vi "WallFollowV4.vi"(4 "Instruction Number":dbl=1.0 format="%#_13g", 6 "Speed Multuiplier":dbl=1.0 format="%#_13g", 7 "Estimated Distnace Travelled (mm)":dbl, 8 "Instruction":T4={"Direction"=enum."Forward", "Relative Tracked Wall"=enum."CW", "Tracking Distance (mm)"=0.0, "Relative Stop Direction"=enum."Dir. of travel", "Stop Distance (mm)"=0.0, "Forward Speed"=0.0, "Action"=enum."None", "Movement"=enum."Normal", "Zone (mm)"=300.0, "Lidar Detection Distance"=300.0}, 9 "Valid":bool[](array[boolean]), 10 "Lidar Angles (deg)":dbl[](array[numeric]), 11 "Lidar Distances (mm)":dbl[](array[numeric])) -> (0 "Direction":T3, 1 "Rotation":dbl, 2 "left/Right":dbl, 3 "Forward/Back":dbl, 5 "Motion Complete":bool)   [LabVIEW 2014]
uses:
  Types/Instruction.ctl
  Types/Direction.ctl
  Types/Action.ctl
  Types/Movement.ctl
panel:
  out "Zone (mm)":dbl
  out "Movement":T1
  out "Relative Tracked Wall":enum16{"None", "CW", "CCW"}(ring)
  out "Mean Distance":dbl[](array[numeric])
  out "Forward Speed (Specified)":dbl
  out "Forward Speed (Clamped)":dbl
  out "Forward Speed (Mult)":dbl
  out "Motor Speed (Chart)":dbl(graph)
  out "Relative Stop Direction":T2(ring)
  out "Left":dbl(slide)
  out "Right":dbl(slide) scale=0.0..500.0
  out "Back":dbl(slide) scale=500.0..0.5
  out "Front":dbl(slide) scale=0.0..500.0
  out "Tracking Distance (mm)":dbl
  out "Stop Distance (mm)":dbl
  out "Forward Speed":dbl
  out "Rotation Speed (Chart)":dbl(graph)
  out "Stop Wall Error":dbl
  out "Wall Rotation Error":dbl
  out "Wall Tracking Error":dbl
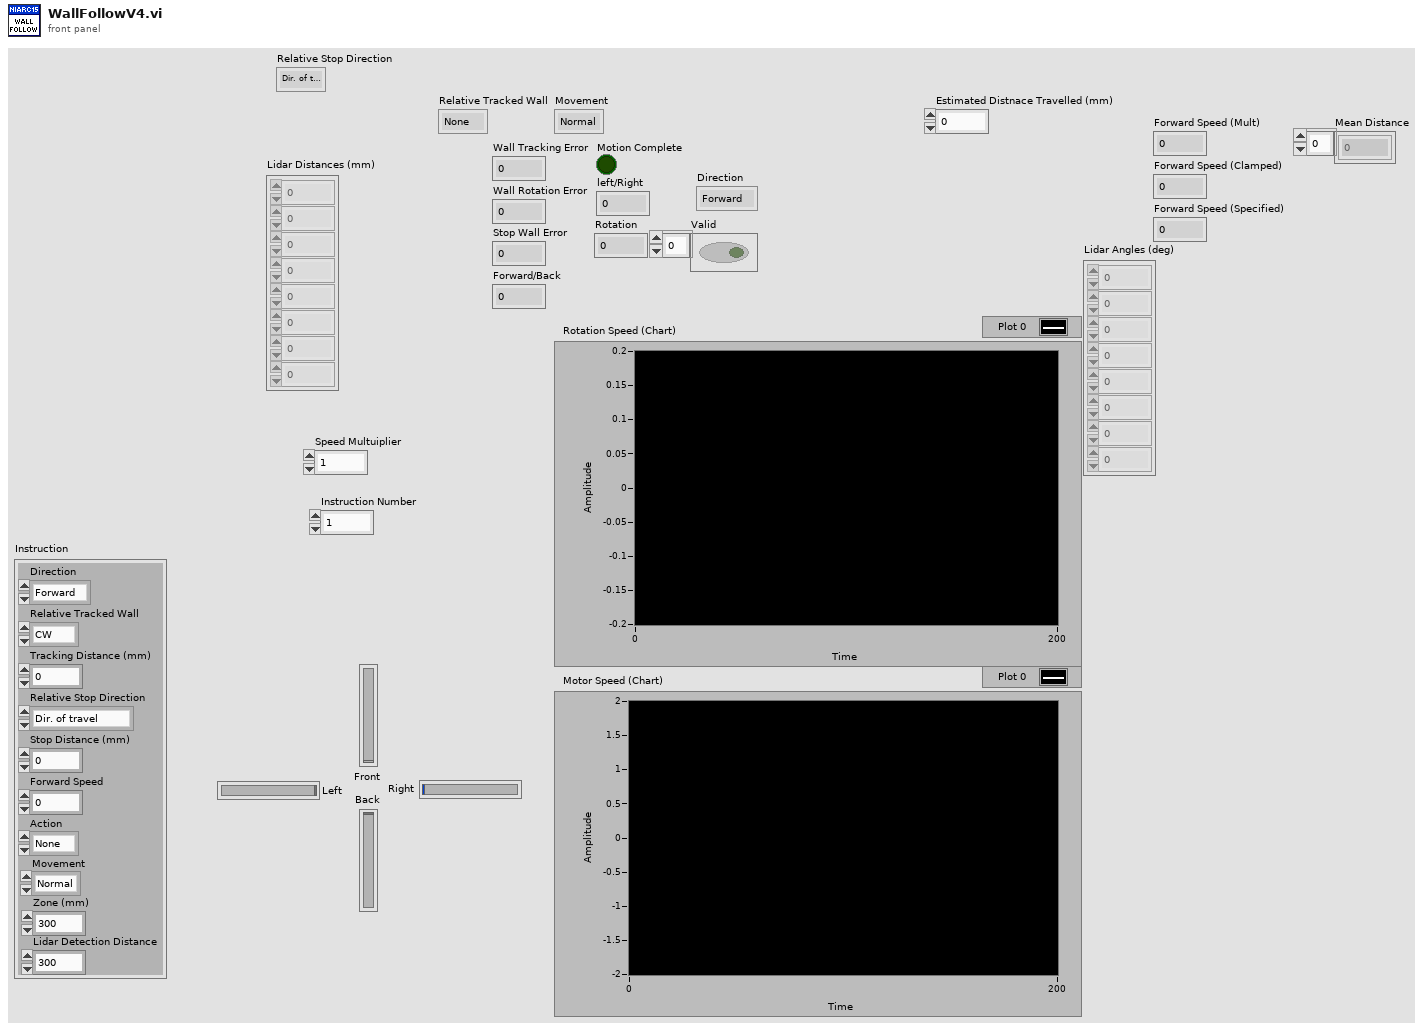
[diagram p1: front panel]
types:
  T1 = typedef "Movement.ctl" = enum16{"Normal", "Align", "Front Right", "Back Right"}
  T2 = enum16{"Dir. of travel", "Counter-dir of travel", "Distance"}
  T3 = typedef "Direction.ctl" = enum16{"Forward", "Left", "Back", "Right"}
  T4 = typedef "Instruction.ctl" = cluster{"Direction":T3, "Relative Tracked Wall":enum16{"None", "CW", "CCW"}, "Tracking Distance (mm)":dbl, "Relative Stop Direction":enum16{"Dir. of travel", "Counter-dir of travel", "Distance"}, "Stop Distance (mm)":dbl, "Forward Speed":dbl, "Action":T5, "Movement":T1, "Zone (mm)":dbl, "Lidar Detection Distance":dbl}
  T5 = typedef "Action.ctl" = enum16{"None", "Wait for Go", "Drop B", "Drop A", "Drop C", "Drop Rear"}
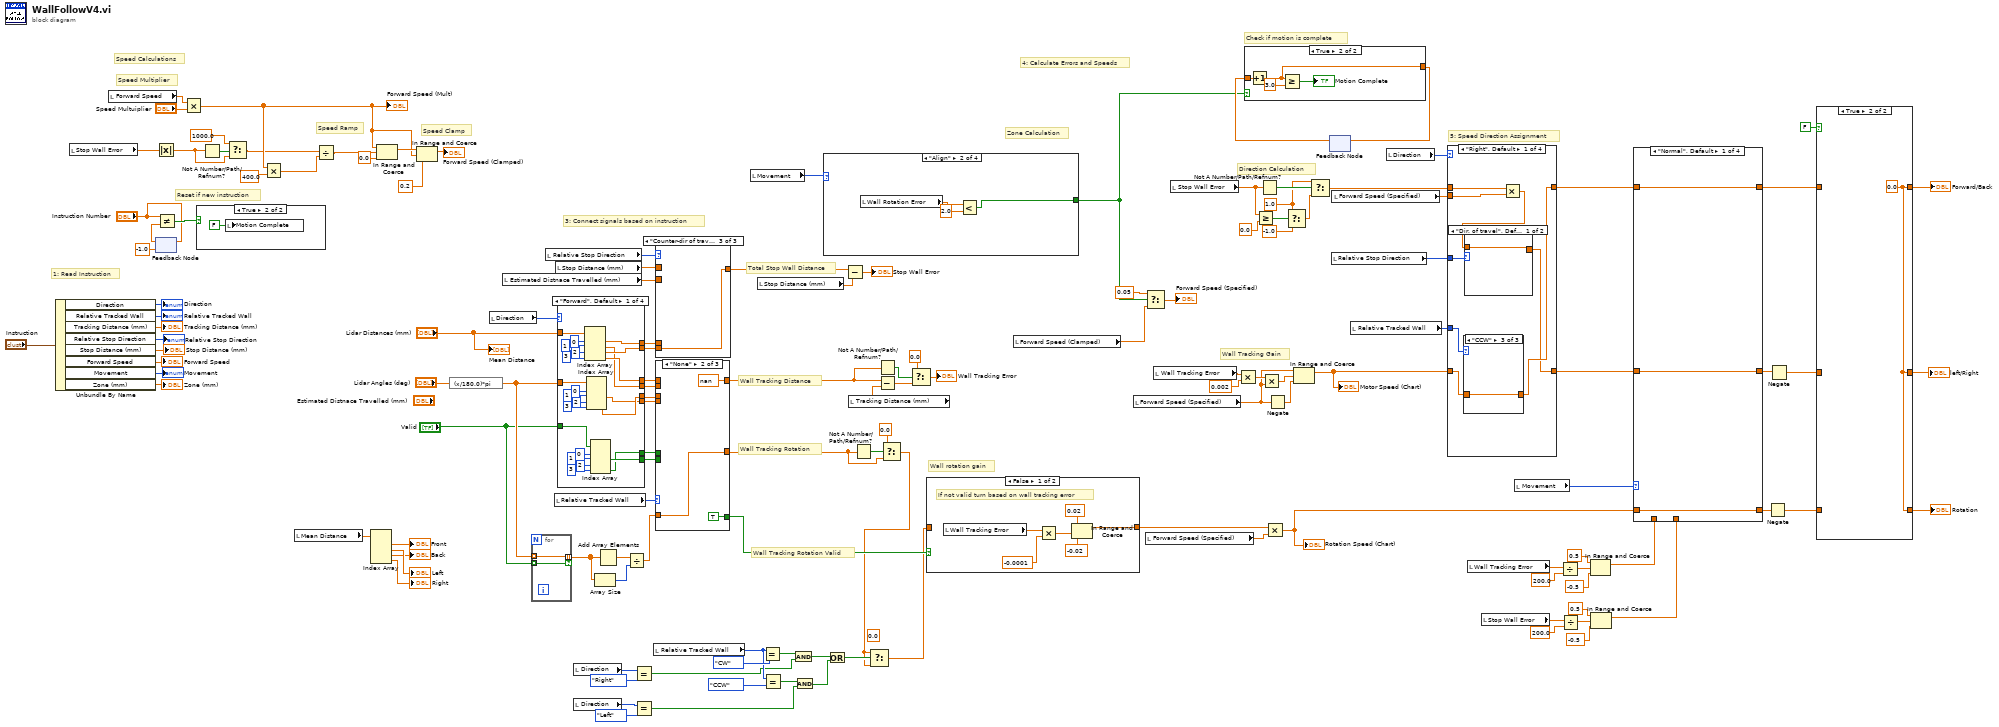
[diagram p0: block diagram]
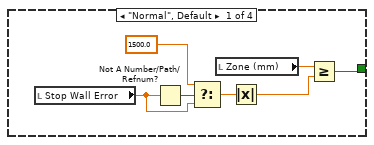
[diagram p4: hidden frame]
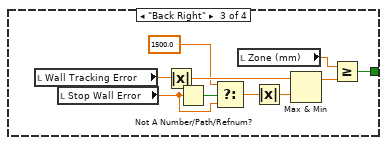
[diagram p5: hidden frame]
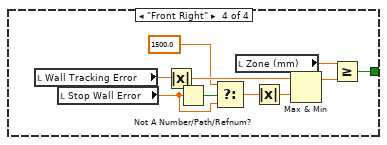
[diagram p6: hidden frame]
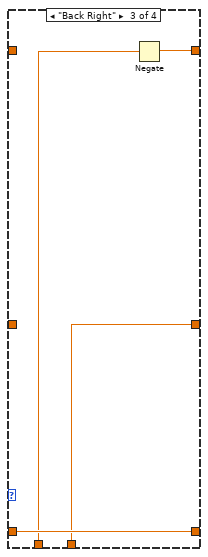
[diagram p8: hidden frame]
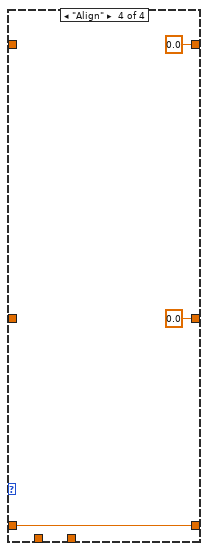
[diagram p9: hidden frame]
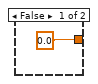
[diagram p10: hidden frame]
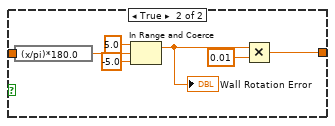
[diagram p11: hidden frame]
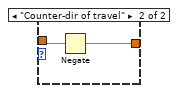
[diagram p12: hidden frame]
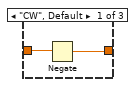
[diagram p13: hidden frame]
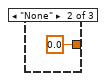
[diagram p14: hidden frame]
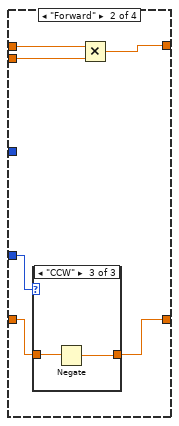
[diagram p15: hidden frame]
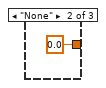
[diagram p17: hidden frame]
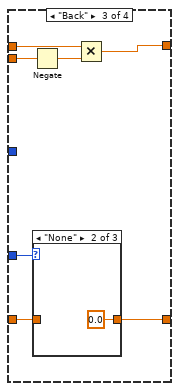
[diagram p18: hidden frame]
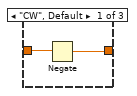
[diagram p19: hidden frame]
diagram:
  (unwired) 0.0 ("t")
  w109 = 1.0 ("t")
  # "Reset if new instruction"
  # "4: Calculate Errors and Speeds"
  # "Wall Tracking Gain"
  # "5: Speed Direction Assignment"
  # "Direction Calculation"
  # "Zone Calculation"
  # "Speed Calculations"
  # "Check if motion is complete"
  # "Speed Clamp"
  # "Speed Ramp"
  # "Speed Multiplier"
  # "Wall rotation gain"
  # "Wall Tracking Rotation Valid"
  # "Wall Tracking Rotation"
  # "Wall Tracking Distance"
  # "Total Stop Wall Distance"
  # "3: Connect signals based on instruction"
  # "1: Read Instruction"
  n1 = Unbundle By Name("Instruction") -> ("Direction"=→"Direction":T3, "Relative Tracked Wall"=→"Relative Tracked Wall":enum16{"None", "CW", "CCW"}, "Tracking Distance (mm)"=→"Tracking Distance (mm)":dbl, "Relative Stop Direction"=→"Relative Stop Direction":T2, "Stop Distance (mm)"=→"Stop Distance (mm)":dbl, "Forward Speed"=→"Forward Speed":dbl, "Movement"=→"Movement":T1, "Zone (mm)"=→"Zone (mm)":dbl)
  n2 = local read "Stop Wall Error"() -> (w28:dbl)
  n3 = local read "Forward Speed"() -> (w91:dbl)
  n4 = feedback-in #1("Instruction Number") -> ()
  n5 = feedback #1(-1.0 ("Instruction Number")) -> (w15:dbl)
  n6 = Absolute Value(x=w28) -> (abs(x)=w27:dbl)
  n7 = Not Equal?(x="Instruction Number", y=w15) -> (x != y?=w13:bool)
  n8 = Multiply(x=w91, y="Speed Multuiplier") -> (x*y=w79:dbl)
  "Forward Speed (Mult)" <- w79
  n9 = case shown="True" w13 {
    frame False {
    }
    frame True {
      n10 = local write "Motion Complete"(FALSE ("Motion Complete")) -> ()
    }
  }
  n11 = Not A Number/Path/Refnum?(number/path/refnum=w27) -> (NaN/Path/Refnum?=w125:bool)
  n12 = Select(t=1000.0, s=w125, f=w27) -> (s? t:f=w10:dbl)
  n13 = Multiply(x=w79, y=400.0) -> (x*y=w78:dbl)
  n14 = local read "Mean Distance"() -> (w69:dbl[])
  n15 = Divide(x=w10, y=w78) -> (x/y=w9:dbl)
  n16 = Index Array(array=w69) -> (element #1=→"Front":dbl, element #2=→"Left":dbl, element #3=→"Back":dbl, element #4=→"Right":dbl)  [unwired: 4 in]
  n17 = In Range and Coerce(upper limit=w79, x=w9, lower limit=0.0) -> (coerced(x)=w124:dbl)  [unwired: 1 out]
  n18 = In Range and Coerce(upper limit=w124, x=w79, lower limit=0.2) -> (coerced(x)=→"Forward Speed (Clamped)":dbl)  [unwired: 1 out]
  n19 = expression code="(x/180.0)*pi" ("degrees to radians")("Lidar Angles (deg)") -> (w8:dbl[])
  n20 = local read "Direction"() -> (w119:T3)
  n21 = local read "Estimated Distnace Travelled (mm)"() -> (w105:dbl)
  n22 = for {
    tunnel: w8 -> [w139] mode=indexing
    tunnel: "Valid" -> [w138] mode=indexing
    tunnel: [w139] -> w6 mode=indexing if=w138
  }
  n23 = local read "Relative Stop Direction"() -> (w118:T2)
  n24 = local read "Relative Tracked Wall"() -> (w117:enum16{"None", "CW", "CCW"})
  n25 = local read "Stop Distance (mm)"() -> (w104:dbl)
  n26 = case shown="\"Forward\", Default" w119 {
    tunnel: "Lidar Distances (mm)" -> [w162 w185 w208 w231]
    tunnel: w8 -> [w153 w176 w199 w222]
    tunnel: [w152 w175 w197 w220] -> w133
    tunnel: [w151 w174 w198 w221] -> w134
    tunnel: [w148 w171 w193 w216] -> w136
    tunnel: [w147 w170 w194 w217] -> w135
    tunnel: [w150 w173 w196 w219] -> w132
    tunnel: [w149 w172 w195 w218] -> w131
    tunnel: "Valid" -> [w142 w165 w188 w211]
    tunnel: [w141 w163 w187 w209] -> w95
    tunnel: [w140 w164 w186 w210] -> w96
    frame "Forward", Default {
      n27 = Index Array(array=w162, index #1=0 ("index"), index #2=1 ("index"), index #3=2 ("index"), index #4=3 ("index")) -> (element #1=w152:dbl, element #2=w149:dbl, element #3=w151:dbl, element #4=w150:dbl)
      n28 = Index Array(array=w153, index #1=0 ("index"), index #2=1 ("index"), index #3=2 ("index"), index #4=3 ("index")) -> (element #2=w147:dbl, element #4=w148:dbl)  [unwired: 2 out]
      n29 = Index Array(array=w142, index #1=0 ("index"), index #2=1 ("index"), index #3=2 ("index"), index #4=3 ("index")) -> (element #2=w141:bool, element #4=w140:bool)  [unwired: 2 out]
    }
    frame "Left" {
      n30 = Index Array(array=w185, index #1=0 ("index"), index #2=1 ("index"), index #3=2 ("index"), index #4=3 ("index")) -> (element #1=w173:dbl, element #2=w175:dbl, element #3=w172:dbl, element #4=w174:dbl)
      n31 = Index Array(array=w176, index #1=0 ("index"), index #2=1 ("index"), index #3=2 ("index"), index #4=3 ("index")) -> (element #1=w171:dbl, element #3=w170:dbl)  [unwired: 2 out]
      n32 = Index Array(array=w165, index #1=0 ("index"), index #2=1 ("index"), index #3=2 ("index"), index #4=3 ("index")) -> (element #1=w164:bool, element #3=w163:bool)  [unwired: 2 out]
    }
    frame "Right" {
      n33 = Index Array(array=w208, index #1=0 ("index"), index #2=1 ("index"), index #3=2 ("index"), index #4=3 ("index")) -> (element #1=w195:dbl, element #2=w198:dbl, element #3=w196:dbl, element #4=w197:dbl)
      n34 = Index Array(array=w199, index #1=0 ("index"), index #2=1 ("index"), index #3=2 ("index"), index #4=3 ("index")) -> (element #1=w194:dbl, element #3=w193:dbl)  [unwired: 2 out]
      n35 = Index Array(array=w188, index #1=0 ("index"), index #2=1 ("index"), index #3=2 ("index"), index #4=3 ("index")) -> (element #1=w187:bool, element #3=w186:bool)  [unwired: 2 out]
    }
    frame "Back" {
      n36 = Index Array(array=w231, index #1=0 ("index"), index #2=1 ("index"), index #3=2 ("index"), index #4=3 ("index")) -> (element #1=w221:dbl, element #2=w219:dbl, element #3=w220:dbl, element #4=w218:dbl)
      n37 = Index Array(array=w222, index #1=0 ("index"), index #2=1 ("index"), index #3=2 ("index"), index #4=3 ("index")) -> (element #2=w216:dbl, element #4=w217:dbl)  [unwired: 2 out]
      n38 = Index Array(array=w211, index #1=0 ("index"), index #2=1 ("index"), index #3=2 ("index"), index #4=3 ("index")) -> (element #2=w210:bool, element #4=w209:bool)  [unwired: 2 out]
    }
  }
  n39 = local read "Direction"() -> (w39:T3)
  n40 = local read "Direction"() -> (w36:T3)
  n41 = Array Size(array=w6) -> (size(s)=w4:i32)
  n42 = Add Array Elements(numeric array=w6) -> (sum=w5:dbl)
  n43 = Divide(x=w5, y=w4) -> (x/y=w3:dbl)
  n44 = Equal?(x=w39, y=Direction."Right") -> (x = y?=w34:bool)
  n45 = Equal?(x=w36, y=Direction."Left") -> (x = y?=w35:bool)
  n46 = local read "Relative Tracked Wall"() -> (w43:enum16{"None", "CW", "CCW"})
  n47 = case shown="\"None\"" w117 {
    tunnel: w136 -> [w234 _ _]
    tunnel: [w234 w235 w240] -> w83
    tunnel: w135 -> [_ _ w240]
    tunnel: w132 -> [w233 _ _]
    tunnel: w131 -> [_ _ w239]
    tunnel: [w233 nan ("Sensor Distances") w239] -> w103
    tunnel: w96 -> [w232 _ _]
    tunnel: w95 -> [_ _ w238]
    tunnel: [w232 TRUE w238] -> w94
    tunnel: w3 -> [_ w235 _]
    frame "CW", Default {
    }
    frame "None" {
    }
    frame "CCW" {
    }
  }
  n48 = case shown="\"Counter-dir of travel\"" w118 {
    tunnel: w134 -> [_ _ w248]
    tunnel: w133 -> [w241 _ _]
    tunnel: [w241 w242 w248] -> w97
    tunnel: w105 -> [_ w247 _]
    tunnel: w104 -> [_ w246 _]
    frame "Dir. of travel", Default {
    }
    frame "Distance" {
      n49 = Absolute Value(x=w247) -> (abs(x)=w243:dbl)
      n50 = Multiply(x=w246, y=2.0) -> (x*y=w244:dbl)
      n51 = Subtract(x=w244, y=w243) -> (x-y=w242:dbl)
    }
    frame "Counter-dir of travel" {
    }
  }
  n52 = local read "Movement"() -> (w57:T1)
  n53 = local read "Stop Distance (mm)"() -> (w75:dbl)
  n54 = Equal?(x=w43, y=enum16{"None", "CW", "CCW"}."CW") -> (x = y?=w40:bool)
  n55 = Equal?(x=w43, y=enum16{"None", "CW", "CCW"}."CCW") -> (x = y?=w41:bool)
  n56 = And(x=w40, y=w34) -> (x .and. y?=w33:bool)
  n57 = And(x=w41, y=w35) -> (x .and. y?=w32:bool)
  n58 = case shown="\"Align\"" w57 {
    tunnel: [w254 w256 w260 w270] -> w30
    frame "Normal", Default {
      n59 = local read "Stop Wall Error"() -> (w251:dbl)
      n60 = Not A Number/Path/Refnum?(number/path/refnum=w251) -> (NaN/Path/Refnum?=w253:bool)
      n61 = Select(t=1500.0, s=w253, f=w251) -> (s? t:f=w252:dbl)
      n62 = local read "Zone (mm)"() -> (w249:dbl)
      n63 = Absolute Value(x=w252) -> (abs(x)=w250:dbl)
      n64 = Greater Or Equal?(x=w249, y=w250) -> (x >= y?=w254:bool)
    }
    frame "Align" {
      n65 = local read "Wall Rotation Error"() -> (w258:dbl)
      n66 = Less?(x=w258, y=2.0) -> (x < y?=w256:bool)
    }
    frame "Back Right" {
      n67 = local read "Wall Tracking Error"() -> (w265:dbl)
      n68 = local read "Stop Wall Error"() -> (w263:dbl)
      n69 = Absolute Value(x=w265) -> (abs(x)=w266:dbl)
      n70 = Not A Number/Path/Refnum?(number/path/refnum=w263) -> (NaN/Path/Refnum?=w262:bool)
      n71 = Select(t=1500.0, s=w262, f=w263) -> (s? t:f=w268:dbl)
      n72 = local read "Zone (mm)"() -> (w259:dbl)
      n73 = Absolute Value(x=w268) -> (abs(x)=w267:dbl)
      n74 = Max & Min(x=w266, y=w267) -> (max(x,y)=w261:dbl)  [unwired: 1 out]
      n75 = Greater Or Equal?(x=w259, y=w261) -> (x >= y?=w260:bool)
    }
    frame "Front Right" {
      n76 = local read "Wall Tracking Error"() -> (w275:dbl)
      n77 = local read "Stop Wall Error"() -> (w273:dbl)
      n78 = Absolute Value(x=w275) -> (abs(x)=w276:dbl)
      n79 = Not A Number/Path/Refnum?(number/path/refnum=w273) -> (NaN/Path/Refnum?=w272:bool)
      n80 = Select(t=1500.0, s=w272, f=w273) -> (s? t:f=w278:dbl)
      n81 = local read "Zone (mm)"() -> (w269:dbl)
      n82 = Absolute Value(x=w278) -> (abs(x)=w277:dbl)
      n83 = Max & Min(x=w276, y=w277) -> (max(x,y)=w271:dbl)  [unwired: 1 out]
      n84 = Greater Or Equal?(x=w269, y=w271) -> (x >= y?=w270:bool)
    }
  }
  n85 = Or(x=w33, y=w32) -> (x .or. y?=w29:bool)
  n86 = Subtract(x=w97, y=w75) -> (x-y=→"Stop Wall Error":dbl)
  n87 = local read "Tracking Distance (mm)"() -> (w116:dbl)
  n88 = Not A Number/Path/Refnum?(number/path/refnum=w83) -> (NaN/Path/Refnum?=w101:bool)
  n89 = Not A Number/Path/Refnum?(number/path/refnum=w103) -> (NaN/Path/Refnum?=w102:bool)
  n90 = Subtract(x=w103, y=w116) -> (x-y=w99:dbl)
  n91 = Select(t=0.0, s=w101, f=w83) -> (s? t:f=w12:dbl)
  n92 = Select(t=w12, s=w29, f=w12) -> (s? t:f=w31:dbl)
  n93 = Select(t=0.0, s=w102, f=w99) -> (s? t:f=→"Wall Tracking Error":dbl)
  n94 = case shown="False" w94 {
    tunnel: [w282 w286] -> w87
    tunnel: w31 -> [_ w287]
    frame False {
      # "If not valid turn based on wall tracking error"
      n95 = local read "Wall Tracking Error"() -> (w279:dbl)
      n96 = Multiply(x=w279, y=-0.0001) -> (x*y=w283:dbl)
      n97 = In Range and Coerce(upper limit=0.02, x=w283, lower limit=-0.02) -> (coerced(x)=w282:dbl)  [unwired: 1 out]
    }
    frame True {
      n98 = expression code="(x/pi)*180.0" ("radians to degrees")(w287) -> (w288:dbl)
      n99 = In Range and Coerce(upper limit=5.0, x=w288, lower limit=-5.0) -> (coerced(x)=w285:dbl)  [unwired: 1 out]
      "Wall Rotation Error" <- w285
      n100 = Multiply(x=w285, y=0.01) -> (x*y=w286:dbl)
    }
  }
  n101 = local read "Forward Speed (Clamped)"() -> (w76:dbl)
  n102 = local read "Forward Speed (Specified)"() -> (w71:dbl)
  n103 = Select(t=0.05, s=w30, f=w76) -> (s? t:f=→"Forward Speed (Specified)":dbl)
  n104 = local read "Forward Speed (Specified)"() -> (w73:dbl)
  n105 = local read "Wall Tracking Error"() -> (w93:dbl)
  n106 = local read "Stop Wall Error"() -> (w112:dbl)
  n107 = Multiply(x=w93, y=0.002) -> (x*y=w86:dbl)
  n108 = Greater Or Equal?(x=w112, y=0.0) -> (x >= y?=w114:bool)
  n109 = Not A Number/Path/Refnum?(number/path/refnum=w112) -> (NaN/Path/Refnum?=w111:bool)
  n110 = Multiply(x=w86, y=w71) -> (x*y=w85:dbl)
  n111 = Multiply(x=w87, y=w73) -> (x*y=w58:dbl)
  "Rotation Speed (Chart)" <- w58
  n112 = Negate(x=w71) -> (-x=w84:dbl)
  n113 = Select(t=w109, s=w114, f=-1.0) -> (s? t:f=w110:dbl)
  n114 = In Range and Coerce(upper limit=w71, x=w85, lower limit=w84) -> (coerced(x)=w70:dbl)  [unwired: 1 out]
  "Motor Speed (Chart)" <- w70
  n115 = Select(t=w109, s=w111, f=w110) -> (s? t:f=w108:dbl)
  n116 = feedback #2() -> (w89:dbl)  [unwired: 1 in]
  n117 = case shown="True" w30 {
    tunnel: w89 -> [_ w296]
    tunnel: [0.0 w294] -> w88
    frame False {
    }
    frame True {
      n118 = Increment(x=w296) -> (x+1=w294:dbl)
      n119 = Greater Or Equal?(x=w294, y=3.0) -> (x >= y?=→"Motion Complete":bool)
    }
  }
  n120 = feedback-in #2(w88) -> ()
  n121 = local read "Relative Stop Direction"() -> (w2:T2)
  n122 = local read "Forward Speed (Specified)"() -> (w72:dbl)
  n123 = local read "Relative Tracked Wall"() -> (w123:enum16{"None", "CW", "CCW"})
  n124 = local read "Direction"() -> (w130:T3)
  n125 = case shown="\"Right\", Default" w130 {
    tunnel: w72 -> [w301 w315 w323 w336]
    tunnel: [w302 w314 w326 w337] -> w60
    tunnel: w70 -> [w304 w317 w328 w339]
    tunnel: [w297 w313 w325 w334] -> w59
    tunnel: w123 -> [w303 w316 w327 w338]
    tunnel: w108 -> [w300 w312 w324 w333]
    tunnel: w2 -> [w299 _ _ _]
    frame "Right", Default {
      n126 = case shown="\"CCW\"" w303 {
        tunnel: w304 -> [w309 _ w311]
        tunnel: [w308 0.0 ("Forward Speed (Specified)") w311] -> w302
        frame "CW", Default {
          n127 = Negate(x=w309) -> (-x=w308:dbl)
        }
        frame "None" {
        }
        frame "CCW" {
        }
      }
      n128 = Multiply(x=w300, y=w301) -> (x*y=w298:dbl)
      n129 = case shown="\"Dir. of travel\", Default" w299 {
        tunnel: w298 -> [w305 w307]
        tunnel: [w305 w306] -> w297
        frame "Dir. of travel", Default {
        }
        frame "Counter-dir of travel" {
          n130 = Negate(x=w307) -> (-x=w306:dbl)
        }
      }
    }
    frame "Forward" {
      n131 = case shown="\"CCW\"" w316 {
        tunnel: w317 -> [w318 _ w321]
        tunnel: [w318 0.0 ("Forward Speed (Specified)") w320] -> w313
        frame "CW", Default {
        }
        frame "None" {
        }
        frame "CCW" {
          n132 = Negate(x=w321) -> (-x=w320:dbl)
        }
      }
      n133 = Multiply(x=w312, y=w315) -> (x*y=w314:dbl)
    }
    frame "Back" {
      n134 = Negate(x=w323) -> (-x=w322:dbl)
      n135 = case shown="\"None\"" w327 {
        tunnel: w328 -> [w330 _ w332]
        tunnel: [w329 0.0 ("Forward Speed (Specified)") w332] -> w325
        frame "CW", Default {
          n136 = Negate(x=w330) -> (-x=w329:dbl)
        }
        frame "None" {
        }
        frame "CCW" {
        }
      }
      n137 = Multiply(x=w324, y=w322) -> (x*y=w326:dbl)
    }
    frame "Left" {
      n138 = case shown="\"None\"" w338 {
        tunnel: w339 -> [w340 w342 _]
        tunnel: [w340 w341 0.0 ("Forward Speed (Specified)")] -> w337
        frame "CW", Default {
        }
        frame "CCW" {
          n139 = Negate(x=w342) -> (-x=w341:dbl)
        }
        frame "None" {
        }
      }
      n140 = Negate(x=w336) -> (-x=w335:dbl)
      n141 = Multiply(x=w333, y=w335) -> (x*y=w334:dbl)
    }
  }
  n142 = local read "Wall Tracking Error"() -> (w56:dbl)
  n143 = local read "Stop Wall Error"() -> (w47:dbl)
  n144 = local read "Movement"() -> (w61:T1)
  n145 = Divide(x=w56, y=200.0) -> (x/y=w53:dbl)
  n146 = Divide(x=w47, y=200.0) -> (x/y=w49:dbl)
  n147 = In Range and Coerce(upper limit=0.5, x=w53, lower limit=-0.5) -> (coerced(x)=w51:dbl)  [unwired: 1 out]
  n148 = In Range and Coerce(upper limit=0.5, x=w49, lower limit=-0.5) -> (coerced(x)=w45:dbl)  [unwired: 1 out]
  n149 = case shown="\"Normal\", Default" w61 {
    tunnel: w60 -> [w346 _ _ _]
    tunnel: [w346 w347 w351 0.0 ("Forward Speed (Specified)")] -> w17
    tunnel: w59 -> [w345 _ _ _]
    tunnel: [w345 w348 w352 0.0 ("Forward Speed (Specified)")] -> w24
    tunnel: w58 -> [w344 w349 w353 w356]
    tunnel: [w344 w349 w353 w356] -> w23
    tunnel: w51 -> [_ w347 w350 _]
    tunnel: w45 -> [_ w348 w352 _]
    frame "Normal", Default {
    }
    frame "Front Right" {
    }
    frame "Back Right" {
      n150 = Negate(x=w350) -> (-x=w351:dbl)
    }
    frame "Align" {
    }
  }
  n151 = Negate(x=w23) -> (-x=w21:dbl)
  n152 = Negate(x=w24) -> (-x=w19:dbl)
  n153 = case shown="True" FALSE {
    tunnel: w21 -> [w359 _]
    tunnel: [w359 w360] -> w20
    tunnel: w19 -> [w358 _]
    tunnel: [w358 w360] -> w18
    tunnel: w17 -> [w357 _]
    tunnel: [w357 w360] -> w16
    frame False {
    }
    frame True {
      w360 = 0.0 ("Forward Speed (Specified)")
    }
  }
  "Forward/Back" <- w16
  "left/Right" <- w18
  "Rotation" <- w20
  "Mean Distance" <- "Lidar Distances (mm)"
